vi "Lookup Source Type.vi"(8 "error in (no error)":errorcluster, 10 "Source Type":string) -> (0 "error out":errorcluster, 3 "Source":refnum<class "BluelinesRedlines Source.lvclass">)   [LabVIEW 2020, in "VolatusGUI.lvlib" / "BluelinesRedlines Source.lvclass"]
uses:
  BluelinesRedlines Source.lvclass
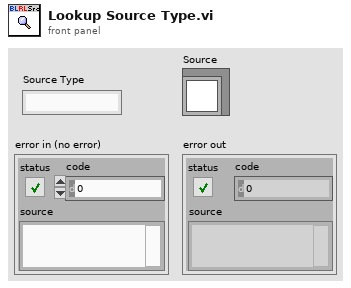
[diagram p1: front panel]
types:
  T1 = map{string, refnum<class "BluelinesRedlines Source.lvclass">}
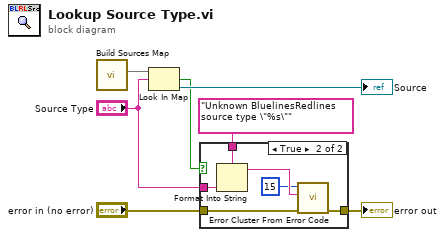
[diagram p0: block diagram]
diagram:
  n1 = call "Build Sources Map.vi"() -> ("Sources"=w7:T1)  [unwired: 11 in]
  n2 = Look In Map(map=w7, key="Source Type") -> (key not found?=w4:bool, value=→"Source":refnum<class "BluelinesRedlines Source.lvclass">)  [unwired: 1 in]
  n3 = case shown="True" w4 {
    tunnel: "error in (no error)" -> [w8 w12]
    tunnel: "Source Type" -> [_ w14]
    tunnel: "Unknown BluelinesRedlines source type \"%s\"" -> [_ w13]
    tunnel: [w8 w9] -> w1
    frame False {
    }
    frame True {
      n4 = Format Into String(format string=w13, w14) -> (resulting string=w11:string)  [unwired: 2 in, 1 out]
      n5 = call <vilib>:"Error Cluster From Error Code.vi"("error in (no error)"=w12, "error message (\"\")"=w11, "error code (0)"=15) -> ("error out"=w9:errorcluster)  [unwired: 6 in]
    }
  }
  "error out" <- w1
